vi "UIinit_CofigYandCurves.vi"(10 "VIref":refnum<vi>, 11 "Language":refnum<vi>) -> ()   [LabVIEW 2015]
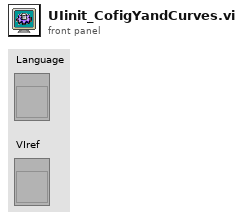
[diagram p1: front panel]
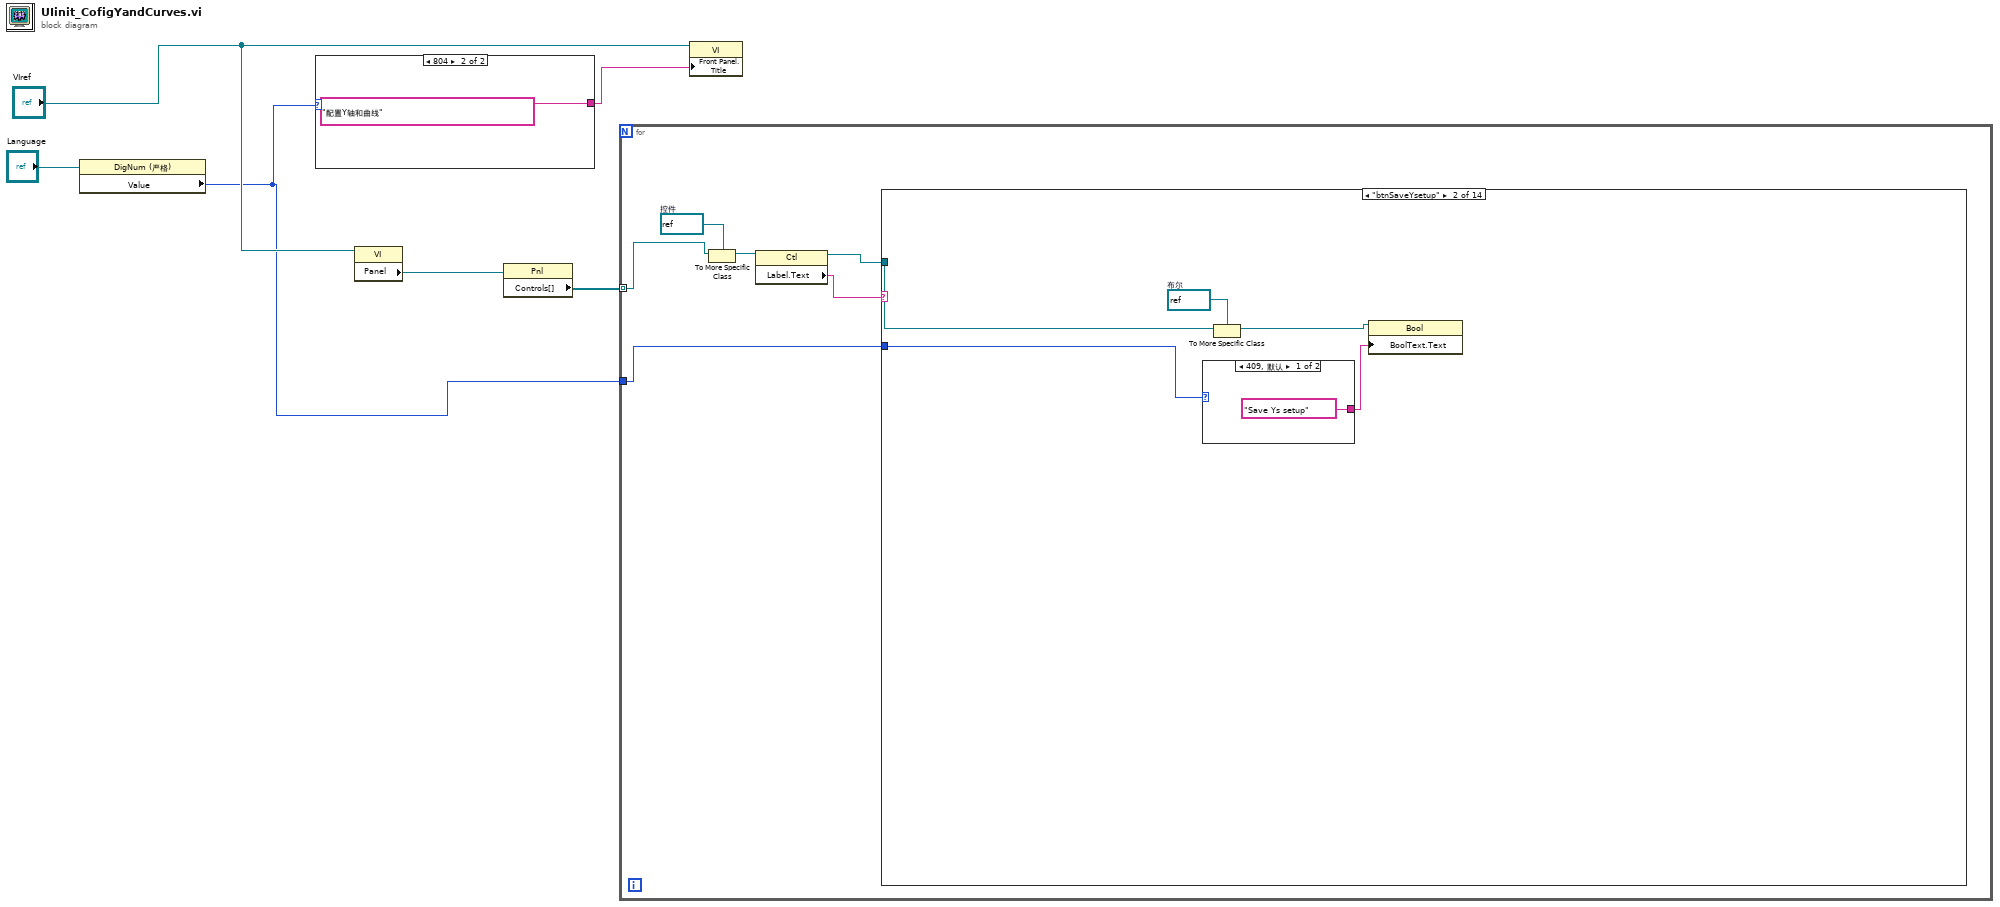
[diagram p0: block diagram]
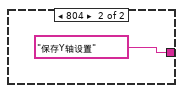
[diagram p3: hidden frame]
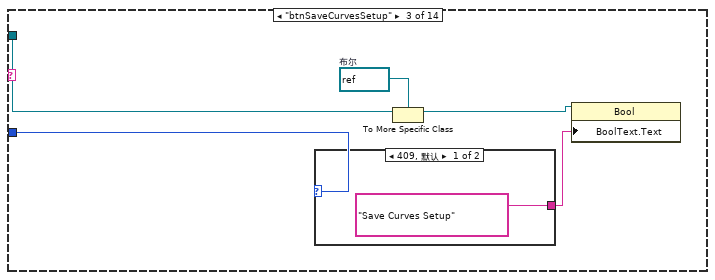
[diagram p4: hidden frame]
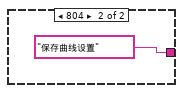
[diagram p5: hidden frame]
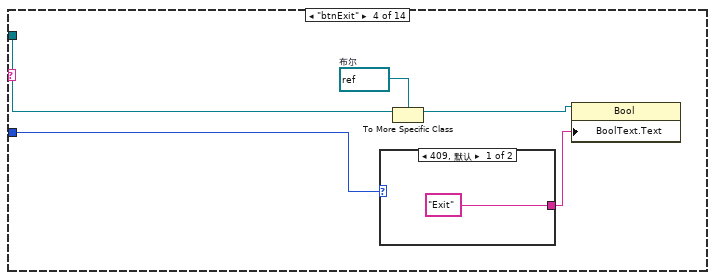
[diagram p6: hidden frame]
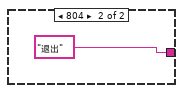
[diagram p7: hidden frame]
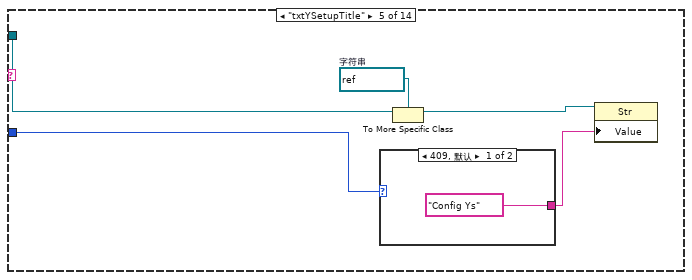
[diagram p8: hidden frame]
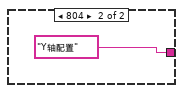
[diagram p9: hidden frame]
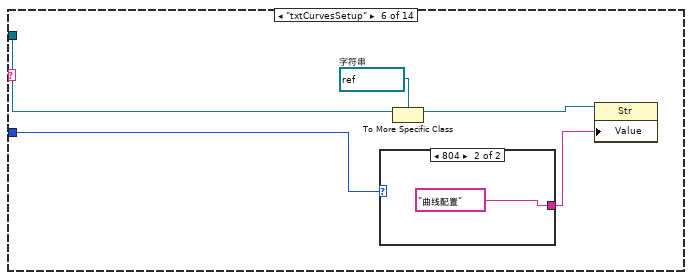
[diagram p10: hidden frame]
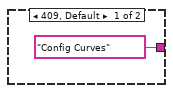
[diagram p11: hidden frame]
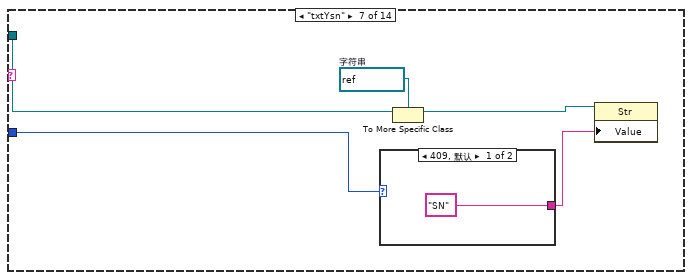
[diagram p12: hidden frame]
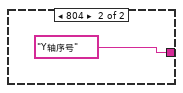
[diagram p13: hidden frame]
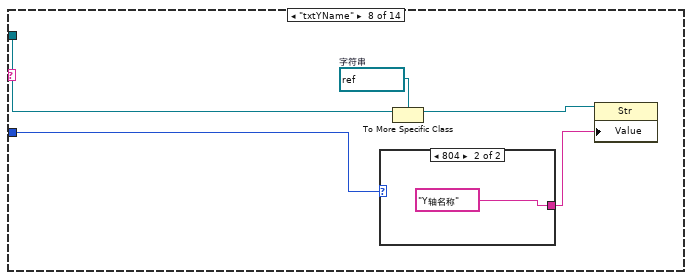
[diagram p14: hidden frame]
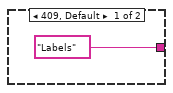
[diagram p15: hidden frame]
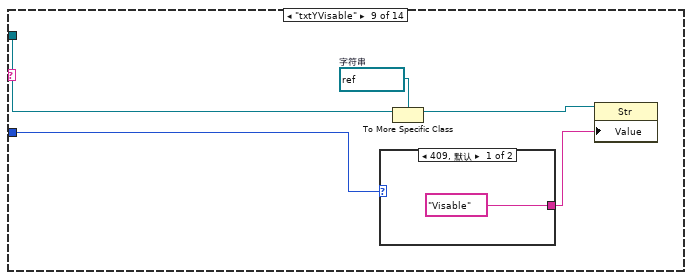
[diagram p16: hidden frame]
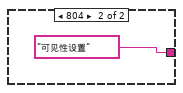
[diagram p17: hidden frame]
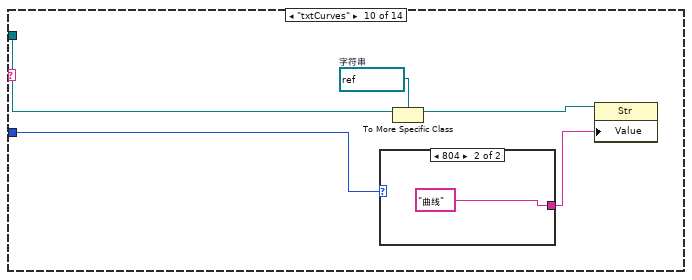
[diagram p18: hidden frame]
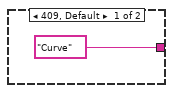
[diagram p19: hidden frame]
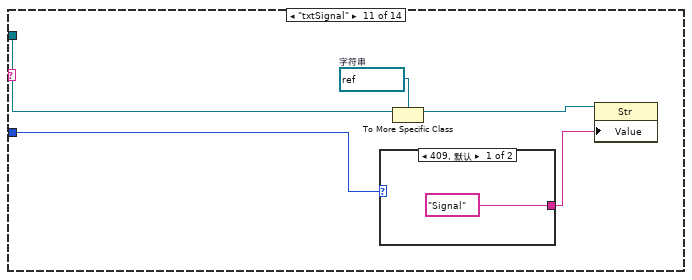
[diagram p20: hidden frame]
diagram:
  n1 = property class="DigNum (严格)"(reference="Language") -> ("Value"=w1:u32)  [unwired: 1 in, 2 out]
  n2 = case shown="804" w1 {
    tunnel: ["Config Y and Curves" "配置Y轴和曲线"] -> w5
    frame 409, Default {
    }
    frame 804 {
    }
  }
  n3 = property class="VI"(reference="VIref") -> ("Panel"=w2:refnum<vi>)  [unwired: 1 in, 2 out]
  n4 = property class="Pnl"(reference=w2) -> ("Controls[]"=w3:refnum<vi>[])  [unwired: 1 in, 2 out]
  n5 = for {
    tunnel: w3 -> [w9] mode=indexing
    tunnel: w1 -> [w10]
    w14 = refnum<vi> refnum  # 控件
    n6 = To More Specific Class(target class=w14, reference=w9) -> (specific class reference=w13:refnum<vi>)  [unwired: 1 in, 1 out]
    n7 = property class="Ctl"(reference=w13) -> (reference out=w11:refnum<vi>, "Label.Text"=w12:string)  [unwired: 1 in, 1 out]
    n8 = case shown="\"btnSaveYsetup\"" w12 {
      tunnel: w11 -> [_ w18 w25 w32 w39 w46 w53 w60 w67 w74 w81 w88 w95 w102]
      tunnel: w10 -> [_ w19 w26 w33 w40 w47 w54 w61 w68 w75 w82 w89 w96 w103]
      frame "假", Default {
      }
      frame "btnSaveYsetup" {
        w17 = refnum<vi> refnum  # 布尔
        n9 = case shown="409, 默认" w19 {
          tunnel: ["Save Ys setup" "保存Y轴设置"] -> w15
          frame 409, Default {
          }
          frame 804 {
          }
        }
        n10 = To More Specific Class(target class=w17, reference=w18) -> (specific class reference=w16:refnum<vi>)  [unwired: 1 in, 1 out]
        n11 = property class="Bool"(reference=w16, "BoolText.Text"=w15) -> ()  [unwired: 1 in, 2 out]
      }
      frame "btnSaveCurvesSetup" {
        w24 = refnum<vi> refnum  # 布尔
        n12 = case shown="409, 默认" w26 {
          tunnel: ["Save Curves Setup" "保存曲线设置"] -> w22
          frame 409, Default {
          }
          frame 804 {
          }
        }
        n13 = To More Specific Class(target class=w24, reference=w25) -> (specific class reference=w23:refnum<vi>)  [unwired: 1 in, 1 out]
        n14 = property class="Bool"(reference=w23, "BoolText.Text"=w22) -> ()  [unwired: 1 in, 2 out]
      }
      frame "btnExit" {
        w31 = refnum<vi> refnum  # 布尔
        n15 = case shown="409, 默认" w33 {
          tunnel: ["Exit" "退出"] -> w29
          frame 409, Default {
          }
          frame 804 {
          }
        }
        n16 = To More Specific Class(target class=w31, reference=w32) -> (specific class reference=w30:refnum<vi>)  [unwired: 1 in, 1 out]
        n17 = property class="Bool"(reference=w30, "BoolText.Text"=w29) -> ()  [unwired: 1 in, 2 out]
      }
      frame "txtYSetupTitle" {
        w38 = refnum<vi> refnum  # 字符串
        n18 = case shown="409, 默认" w40 {
          tunnel: ["Config Ys" "Y轴配置"] -> w36
          frame 409, Default {
          }
          frame 804 {
          }
        }
        n19 = To More Specific Class(target class=w38, reference=w39) -> (specific class reference=w37:refnum<vi>)  [unwired: 1 in, 1 out]
        n20 = property class="Str"(reference=w37, "Value"=w36) -> ()  [unwired: 1 in, 2 out]
      }
      frame "txtCurvesSetup" {
        w45 = refnum<vi> refnum  # 字符串
        n21 = case shown="804" w47 {
          tunnel: ["Config Curves" "曲线配置"] -> w43
          frame 409, Default {
          }
          frame 804 {
          }
        }
        n22 = To More Specific Class(target class=w45, reference=w46) -> (specific class reference=w44:refnum<vi>)  [unwired: 1 in, 1 out]
        n23 = property class="Str"(reference=w44, "Value"=w43) -> ()  [unwired: 1 in, 2 out]
      }
      frame "txtYsn" {
        w52 = refnum<vi> refnum  # 字符串
        n24 = case shown="409, 默认" w54 {
          tunnel: ["SN" "Y轴序号"] -> w50
          frame 409, Default {
          }
          frame 804 {
          }
        }
        n25 = To More Specific Class(target class=w52, reference=w53) -> (specific class reference=w51:refnum<vi>)  [unwired: 1 in, 1 out]
        n26 = property class="Str"(reference=w51, "Value"=w50) -> ()  [unwired: 1 in, 2 out]
      }
      frame "txtYName" {
        w59 = refnum<vi> refnum  # 字符串
        n27 = case shown="804" w61 {
          tunnel: ["Labels" "Y轴名称"] -> w57
          frame 409, Default {
          }
          frame 804 {
          }
        }
        n28 = To More Specific Class(target class=w59, reference=w60) -> (specific class reference=w58:refnum<vi>)  [unwired: 1 in, 1 out]
        n29 = property class="Str"(reference=w58, "Value"=w57) -> ()  [unwired: 1 in, 2 out]
      }
      frame "txtYVisable" {
        w66 = refnum<vi> refnum  # 字符串
        n30 = case shown="409, 默认" w68 {
          tunnel: ["Visable" "可见性设置"] -> w64
          frame 409, Default {
          }
          frame 804 {
          }
        }
        n31 = To More Specific Class(target class=w66, reference=w67) -> (specific class reference=w65:refnum<vi>)  [unwired: 1 in, 1 out]
        n32 = property class="Str"(reference=w65, "Value"=w64) -> ()  [unwired: 1 in, 2 out]
      }
      frame "txtCurves" {
        w73 = refnum<vi> refnum  # 字符串
        n33 = case shown="804" w75 {
          tunnel: ["Curve" "曲线"] -> w71
          frame 409, Default {
          }
          frame 804 {
          }
        }
        n34 = To More Specific Class(target class=w73, reference=w74) -> (specific class reference=w72:refnum<vi>)  [unwired: 1 in, 1 out]
        n35 = property class="Str"(reference=w72, "Value"=w71) -> ()  [unwired: 1 in, 2 out]
      }
      frame "txtSignal" {
        w80 = refnum<vi> refnum  # 字符串
        n36 = case shown="409, 默认" w82 {
          tunnel: ["Signal" "信号名"] -> w78
          frame 409, Default {
          }
          frame 804 {
          }
        }
        n37 = To More Specific Class(target class=w80, reference=w81) -> (specific class reference=w79:refnum<vi>)  [unwired: 1 in, 1 out]
        n38 = property class="Str"(reference=w79, "Value"=w78) -> ()  [unwired: 1 in, 2 out]
      }
      frame "txtUnit" {
        w87 = refnum<vi> refnum  # 字符串
        n39 = case shown="804" w89 {
          tunnel: ["Unit" "单位"] -> w85
          frame 409, Default {
          }
          frame 804 {
          }
        }
        n40 = To More Specific Class(target class=w87, reference=w88) -> (specific class reference=w86:refnum<vi>)  [unwired: 1 in, 1 out]
        n41 = property class="Str"(reference=w86, "Value"=w85) -> ()  [unwired: 1 in, 2 out]
      }
      frame "txtRename" {
        w94 = refnum<vi> refnum  # 字符串
        n42 = case shown="409, 默认" w96 {
          tunnel: ["Rename" "自定曲线名"] -> w92
          frame 409, Default {
          }
          frame 804 {
          }
        }
        n43 = To More Specific Class(target class=w94, reference=w95) -> (specific class reference=w93:refnum<vi>)  [unwired: 1 in, 1 out]
        n44 = property class="Str"(reference=w93, "Value"=w92) -> ()  [unwired: 1 in, 2 out]
      }
      frame "txtYlink" {
        w101 = refnum<vi> refnum  # 字符串
        n45 = case shown="804" w103 {
          tunnel: ["Y Linked" "关联Y轴"] -> w99
          frame 409, Default {
          }
          frame 804 {
          }
        }
        n46 = To More Specific Class(target class=w101, reference=w102) -> (specific class reference=w100:refnum<vi>)  [unwired: 1 in, 1 out]
        n47 = property class="Str"(reference=w100, "Value"=w99) -> ()  [unwired: 1 in, 2 out]
      }
    }
  }
  n48 = property class="VI"(reference="VIref", "Front Panel.Title"=w5) -> ()  [unwired: 1 in, 2 out]
